vi "myRIO v1.0 Read I2C.vi"(4 "Keep Bus Busy":bool, 6 "Slave Address (7-bit)":u8, 7 "Timeout ms (1000)":i32=1000, 8 "Error In (No Error)":errorcluster, 9 "Bytes to Read":u32, 10 "Channel":T1, 11 "myRIO Ref In":T2) -> (0 "error out":errorcluster, 2 "Data Read":u8[](array[numeric]), 3 "myRIO Ref Out":T2)   [LabVIEW 2021]
uses:
  <vilib>/myRIO/Common/Instrument Driver Framework/Utilities/typedefs/myRIO v1.0 Reference.ctl
  <vilib>/myRIO/Common/Instrument Driver Framework/Utilities/typedefs/Generic FPGA Reference.ctl
  <vilib>/myRIO/Common/Instrument Driver Framework/myRIO v1.0/I2C/typedefs/I2C Channels Enum.ctl
  <vilib>/myRIO/Common/Instrument Driver Framework/myRIO v1.0/I2C/typedefs/I2C Channels FPGA Reference.ctl
  <vilib>/rvi/errors/niLvFpgaAdjustHostInterfaceError.vi
  <vilib>/rvi/interface/nirviReadWriteControl/nirviReadWriteControl.xnode
  <vilib>/rvi/interface/Simulation/niFpgaSimulationCallBeginRW.vi
  NiFpgaLv.dll
panel:
  # "This VI writes an array of data to the SPI Data Out register (SPIn.SPDO) and reads an array of data from the SPI Data In register (SPIn.SPDI) for a particular SPI channel (n). The data is written/read one value at a time. Please see Block Diagram for details."
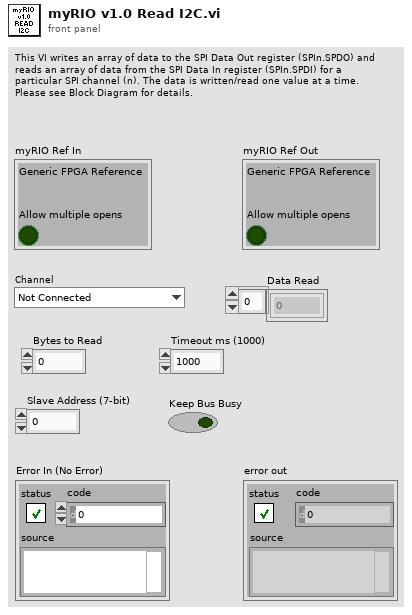
[diagram p1: front panel]
types:
  T1 = typedef "I2C Channels Enum.ctl" = enum16{"Not Connected", "A/I2C", "B/I2C", "I2C/I2C"}
  T2 = typedef "myRIO v1.0 Reference.ctl" = cluster{"Generic FPGA Reference":T3, "Allow multiple opens":bool}
  T3 = typedef "Generic FPGA Reference.ctl" = refnum<k20>
  T4 = typedef "I2C Channels FPGA Reference.ctl" = refnum<k20>
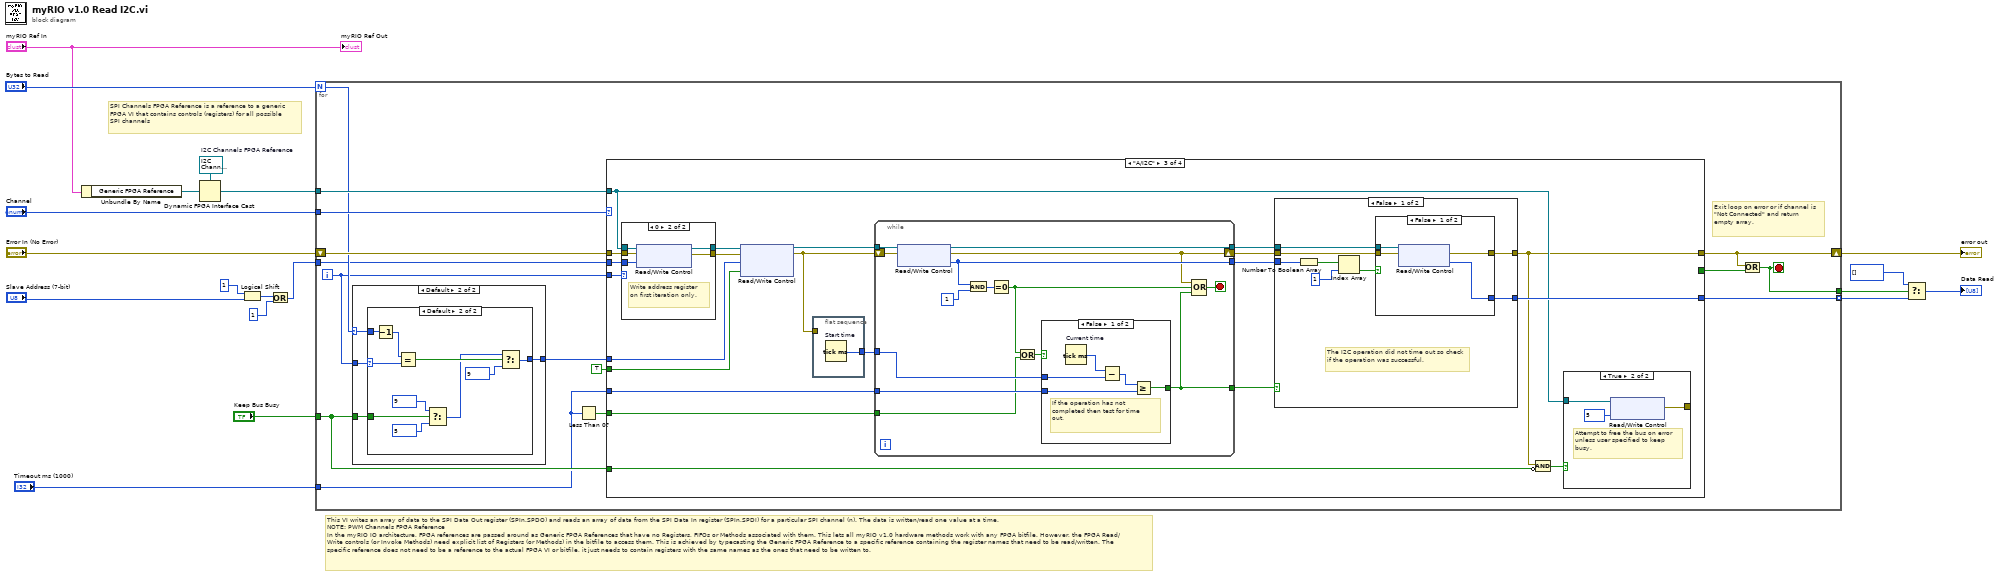
[diagram p0: block diagram]
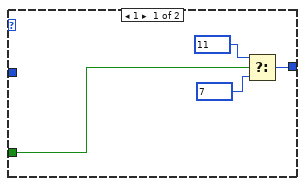
[diagram p2: hidden frame]
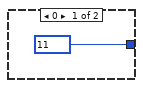
[diagram p3: hidden frame]
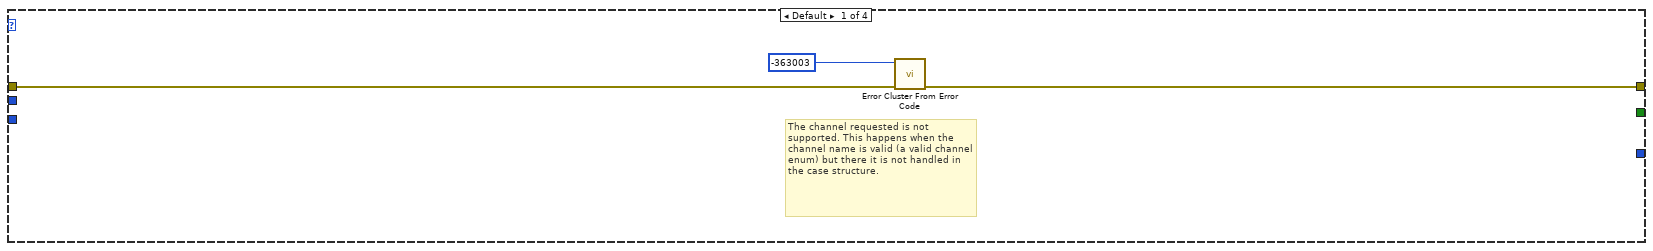
[diagram p4: hidden frame]
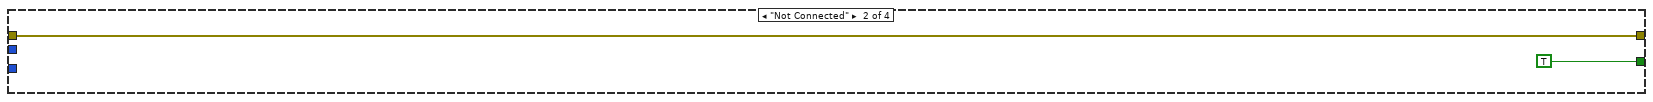
[diagram p5: hidden frame]
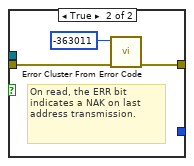
[diagram p6: hidden frame]
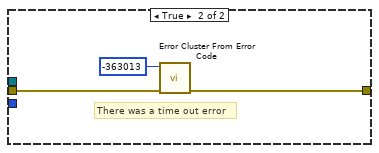
[diagram p7: hidden frame]
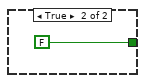
[diagram p10: hidden frame]
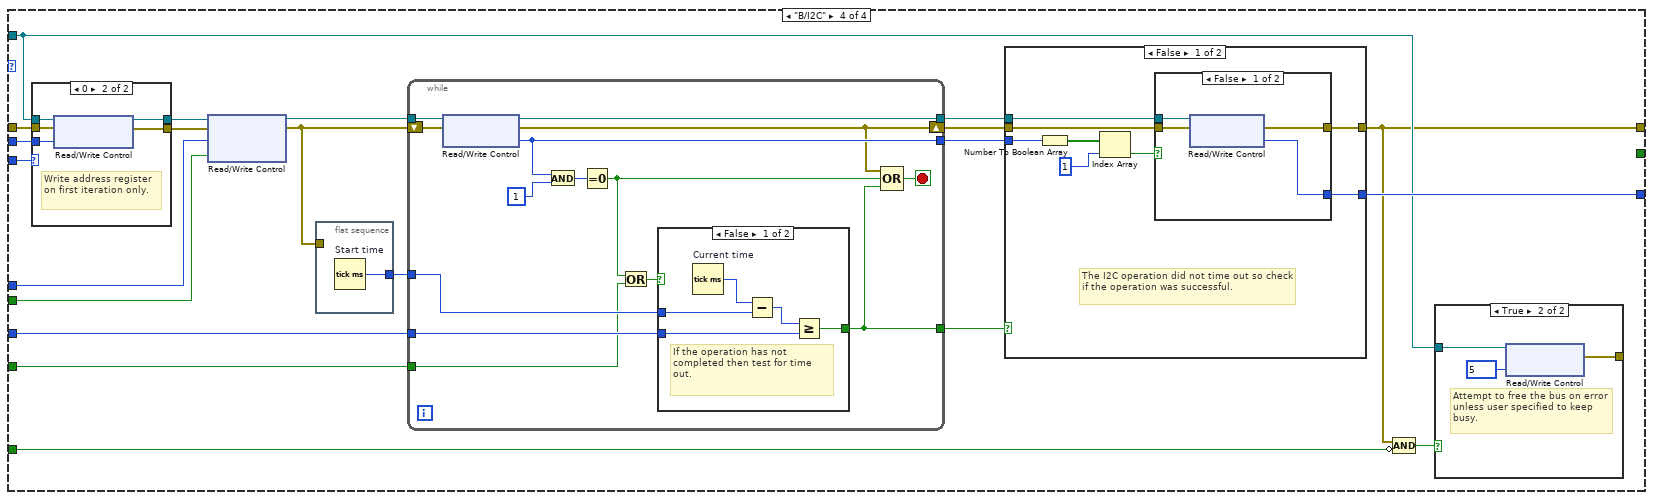
[diagram p11: hidden frame]
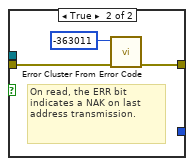
[diagram p12: hidden frame]
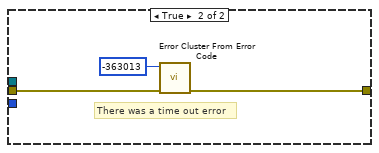
[diagram p13: hidden frame]
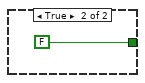
[diagram p16: hidden frame]
diagram:
  w17 = T4 refnum  # I2C Channels FPGA Reference
  # "This VI writes an array of data to the SPI Data Out register (SPIn.SPDO) and reads an array of data from the SPI Data In register (SPIn.SPDI) for a particular SPI channel (n). The data is written/read one value at a time.\nNOTE: PWM Channels FPGA Reference\nIn the myRIO IO architecture, FPGA references are passed around as Generic FPGA References that have no Registers, FIFOs or Methods associated with them. This lets all myRIO v1.0 hardware methods work with any FPGA bitfile. However, the FPGA Read/Write controls (or Invoke Methods) need explicit list of Registers (or Methods) in the bitfile to access them. This is achieved by typecasting the Generic FPGA Reference to a specific reference containing the register names that need to be read/written. The specific reference does not need to be a reference to the actual FPGA VI or bitfile, it just needs to contain registers with the same names as the ones that need to be written to."
  # "SPI Channels FPGA Reference is a reference to a generic FPGA VI that contains controls (registers) for all possible SPI channels"
  n1 = Unbundle By Name("myRIO Ref In") -> ("Generic FPGA Reference"=w1:T3)
  n2 = Dynamic FPGA Interface Cast(Session In=w17, Type=w1) -> (Session Out=w5:T4)
  n3 = Logical Shift(y=i8 1, x="Slave Address (7-bit)") -> (x << y=w16:u8)
  n4 = Or(x=w16, y=u8 1) -> (x .or. y?=w4:u8)
  n5 = for {
    N: "Bytes to Read" -> [w29]
    tunnel: "Channel" -> [w33]
    shift-right: [w24] -> w9
    shift-left: "Error In (No Error)" -> [w34]
    tunnel: w5 -> [w32]
    tunnel: [w28] -> w7 mode=indexing
    tunnel: [w22] -> w8
    tunnel: "Keep Bus Busy" -> [w25]
    tunnel: w4 -> [w27]
    tunnel: "Timeout ms (1000)" -> [w21]
    i -> [w26]
    stop <- w22 stop-if-true
    # "Exit loop on error or if channel is \"Not Connected\" and return empty array."
    n6 = case shown="Default" w29 {
      selector: w29 -> [_ w40]
      tunnel: [w38 w41] -> w30
      tunnel: w26 -> [_ w42]
      tunnel: w25 -> [w36 w39]
      frame 1 {
        n7 = Select(t=u8 11 ("y"), s=w36, f=u8 7 ("y")) -> (s? t:f=w38:u8)
      }
      frame Default {
        n8 = case shown="Default" w42 {
          selector: w42 -> [_ w51]
          tunnel: [u8 11 ("y") w49] -> w41
          tunnel: w40 -> [_ w53]
          tunnel: w39 -> [_ w46]
          frame 0 {
          }
          frame Default {
            n9 = Decrement(x=w53) -> (x-1=w52:i32)
            n10 = Equal?(x=w52, y=w51) -> (x = y?=w50:bool)
            n11 = Select(t=u8 9 ("y"), s=w46, f=u8 5 ("y")) -> (s? t:f=w45:u8)
            n12 = Select(t=w45, s=w50, f=u8 9 ("y")) -> (s? t:f=w49:u8)
          }
        }
      }
    }
    n13 = Less Than 0?(x=w21) -> (x < 0?=w20:bool)
    n14 = case shown="\"A/I2C\"" w33 {
      tunnel: w34 -> [w55 w58 w70 w140]
      tunnel: [w54 w58 w65 w135] -> w24
      tunnel: w32 -> [_ _ w67 w137]
      tunnel: w30 -> [_ _ w79 w149]
      tunnel: TRUE ("I2C0.GO") -> [_ _ w78 w148]
      tunnel: [_ _ w74 w144] -> w28
      tunnel: [_ TRUE _ _] -> w23
      tunnel: w27 -> [_ _ w69 w139]
      tunnel: w26 -> [_ _ w68 w138]
      tunnel: w25 -> [_ _ w66 w136]
      tunnel: w21 -> [_ _ w61 w131]
      tunnel: w20 -> [_ _ w60 w130]
      frame Default {
        # "The channel requested is not supported. This happens when the channel name is valid (a valid channel enum) but there it is not handled in the case structure."
        n15 = call <vilib>:"Error Cluster From Error Code.vi"("error in (no error)"=w55, "error code (0)"=-363003) -> ("error out"=w54:errorcluster)  [unwired: 7 in]
      }
      frame "Not Connected" {
      }
      frame "A/I2C" {
        n16 = case shown="0" w68 {
          tunnel: [w103 w108] -> w72
          tunnel: [w102 w107] -> w71
          tunnel: w67 -> [w103 w106]
          tunnel: w70 -> [w102 w105]
          tunnel: w69 -> [_ w104]
          frame Default {
          }
          frame 0 {
            # "Write address register on first iteration only."
            n17 = xnode "Read/Write Control"("FPGA VI Reference In"=w106, "error in"=w105, "I2C.A.ADDR"=w104) -> ("FPGA VI Reference Out"=w108:T4, "error out"=w107:errorcluster)
          }
        }
        n18 = xnode "Read/Write Control"("FPGA VI Reference In"=w72, "error in"=w71, "I2C.A.CNTL"=w79, "I2C.A.GO"=w78) -> ("FPGA VI Reference Out"=w77:T4, "error out"=w59:errorcluster)
        n19 = flat-sequence {
          tunnel: [w80] -> w63
          tunnel: w59 -> [_]
          frame #0 {
            n20 = Tick Count (ms) "Start time"() -> (millisecond timer value=w80:u32)
          }
        }
        n21 = while {
          tunnel: w77 -> [w121]
          shift-right: [w115] -> w76
          shift-left: w59 -> [w122]
          tunnel: [w117] -> w75
          tunnel: [w116] -> w73
          tunnel: w63 -> [w114]
          tunnel: [w113] -> w62
          tunnel: w61 -> [w112]
          tunnel: w60 -> [w110]
          stop <- w118 stop-if-true
          n22 = xnode "Read/Write Control"("FPGA VI Reference In"=w121, "error in"=w122) -> ("FPGA VI Reference Out"=w116:T4, "error out"=w115:errorcluster, "I2C.A.STAT"=w117:u8)
          n23 = And(x=w117, y=u8 1) -> (x .and. y?=w119:u8)
          n24 = Equal To 0?(x=w119) -> (x = 0?=w109:bool)
          n25 = Or(x=w109, y=w110) -> (x .or. y?=w111:bool)
          n26 = case shown="False" w111 {
            tunnel: w114 -> [w125 _]
            tunnel: [w124 FALSE] -> w113
            tunnel: w112 -> [w123 _]
            frame False {
              # "If the operation has not completed then test for time out."
              n27 = Tick Count (ms) "Current time"() -> (millisecond timer value=w126:u32)
              n28 = Subtract(x=w126, y=w125) -> (x-y=w127:u32)
              n29 = Greater Or Equal?(x=w127, y=w123) -> (x >= y?=w124:bool)
            }
            frame True {
            }
          }
          n30 = Compound Arithmetic op=OR(w115, w109, w113) -> (w118:bool)
        }
        n31 = case shown="False" w62 {
          tunnel: w76 -> [w88 w97]
          tunnel: w75 -> [w87 _]
          tunnel: [w83 _] -> w74
          tunnel: w73 -> [w82 _]
          tunnel: [w81 w96] -> w65
          frame False {
            # "The I2C operation did not time out so check if the operation was successful."
            n32 = Number To Boolean Array(number=w87) -> (Boolean array=w86:bool[])
            n33 = Index Array(array=w86, index=1) -> (element=w85:bool)
            n34 = case shown="False" w85 {
              tunnel: w88 -> [w90 w93]
              tunnel: [w91 w95] -> w81
              tunnel: [w92 _] -> w83
              tunnel: w82 -> [w89 _]
              frame False {
                n35 = xnode "Read/Write Control"("FPGA VI Reference In"=w89, "error in"=w90) -> ("error out"=w91:errorcluster, "I2C.A.DATI"=w92:u8)  [unwired: 1 out]
              }
              frame True {
                # "On read, the ERR bit indicates a NAK on last address transmission."
                n36 = call <vilib>:"Error Cluster From Error Code.vi"("error in (no error)"=w93, "error code (0)"=-363011) -> ("error out"=w95:errorcluster)  [unwired: 7 in]
              }
            }
          }
          frame True {
            # "There was a time out error"
            n37 = call <vilib>:"Error Cluster From Error Code.vi"("error in (no error)"=w97, "error code (0)"=-363013) -> ("error out"=w96:errorcluster)  [unwired: 7 in]
          }
        }
        n38 = Compound Arithmetic op=AND(w65, invert w66) -> (w64:bool)
        n39 = case shown="True" w64 {
          tunnel: w67 -> [_ w101]
          tunnel: [_ w99] -> _
          frame False {
          }
          frame True {
            # "Attempt to free the bus on error unless user specified to keep busy."
            n40 = xnode "Read/Write Control"("FPGA VI Reference In"=w101, "I2C.A.CNTL"=u8 5 ("I2C.C_0.CNTL")) -> ("error out"=w99:errorcluster)  [unwired: 1 in, 1 out]
          }
        }
      }
      frame "B/I2C" {
        n41 = case shown="0" w138 {
          tunnel: [w173 w178] -> w142
          tunnel: [w172 w177] -> w141
          tunnel: w137 -> [w173 w176]
          tunnel: w140 -> [w172 w175]
          tunnel: w139 -> [_ w174]
          frame Default {
          }
          frame 0 {
            # "Write address register on first iteration only."
            n42 = xnode "Read/Write Control"("FPGA VI Reference In"=w176, "error in"=w175, "I2C.B.ADDR"=w174) -> ("FPGA VI Reference Out"=w178:T4, "error out"=w177:errorcluster)
          }
        }
        n43 = xnode "Read/Write Control"("FPGA VI Reference In"=w142, "error in"=w141, "I2C.B.CNTL"=w149, "I2C.B.GO"=w148) -> ("FPGA VI Reference Out"=w147:T4, "error out"=w129:errorcluster)
        n44 = flat-sequence {
          tunnel: [w150] -> w133
          tunnel: w129 -> [_]
          frame #0 {
            n45 = Tick Count (ms) "Start time"() -> (millisecond timer value=w150:u32)
          }
        }
        n46 = while {
          tunnel: w147 -> [w191]
          shift-right: [w185] -> w146
          shift-left: w129 -> [w192]
          tunnel: [w187] -> w145
          tunnel: [w186] -> w143
          tunnel: w133 -> [w184]
          tunnel: [w183] -> w132
          tunnel: w131 -> [w182]
          tunnel: w130 -> [w180]
          stop <- w188 stop-if-true
          n47 = xnode "Read/Write Control"("FPGA VI Reference In"=w191, "error in"=w192) -> ("FPGA VI Reference Out"=w186:T4, "error out"=w185:errorcluster, "I2C.B.STAT"=w187:u8)
          n48 = And(x=w187, y=u8 1) -> (x .and. y?=w189:u8)
          n49 = Equal To 0?(x=w189) -> (x = 0?=w179:bool)
          n50 = Or(x=w179, y=w180) -> (x .or. y?=w181:bool)
          n51 = case shown="False" w181 {
            tunnel: w184 -> [w195 _]
            tunnel: [w194 FALSE] -> w183
            tunnel: w182 -> [w193 _]
            frame False {
              # "If the operation has not completed then test for time out."
              n52 = Tick Count (ms) "Current time"() -> (millisecond timer value=w196:u32)
              n53 = Subtract(x=w196, y=w195) -> (x-y=w197:u32)
              n54 = Greater Or Equal?(x=w197, y=w193) -> (x >= y?=w194:bool)
            }
            frame True {
            }
          }
          n55 = Compound Arithmetic op=OR(w185, w179, w183) -> (w188:bool)
        }
        n56 = case shown="False" w132 {
          tunnel: w146 -> [w158 w167]
          tunnel: w145 -> [w157 _]
          tunnel: [w153 _] -> w144
          tunnel: w143 -> [w152 _]
          tunnel: [w151 w166] -> w135
          frame False {
            # "The I2C operation did not time out so check if the operation was successful."
            n57 = Number To Boolean Array(number=w157) -> (Boolean array=w156:bool[])
            n58 = Index Array(array=w156, index=1) -> (element=w155:bool)
            n59 = case shown="False" w155 {
              tunnel: w158 -> [w160 w163]
              tunnel: [w161 w165] -> w151
              tunnel: [w162 _] -> w153
              tunnel: w152 -> [w159 _]
              frame False {
                n60 = xnode "Read/Write Control"("FPGA VI Reference In"=w159, "error in"=w160) -> ("error out"=w161:errorcluster, "I2C.B.DATI"=w162:u8)  [unwired: 1 out]
              }
              frame True {
                # "On read, the ERR bit indicates a NAK on last address transmission."
                n61 = call <vilib>:"Error Cluster From Error Code.vi"("error in (no error)"=w163, "error code (0)"=-363011) -> ("error out"=w165:errorcluster)  [unwired: 7 in]
              }
            }
          }
          frame True {
            # "There was a time out error"
            n62 = call <vilib>:"Error Cluster From Error Code.vi"("error in (no error)"=w167, "error code (0)"=-363013) -> ("error out"=w166:errorcluster)  [unwired: 7 in]
          }
        }
        n63 = Compound Arithmetic op=AND(w135, invert w136) -> (w134:bool)
        n64 = case shown="True" w134 {
          tunnel: w137 -> [_ w171]
          tunnel: [_ w169] -> _
          frame False {
          }
          frame True {
            # "Attempt to free the bus on error unless user specified to keep busy."
            n65 = xnode "Read/Write Control"("FPGA VI Reference In"=w171, "I2C.B.CNTL"=u8 5 ("I2C.C_0.CNTL")) -> ("error out"=w169:errorcluster)  [unwired: 1 in, 1 out]
          }
        }
      }
    }
    n66 = Or(x=w24, y=w23) -> (x .or. y?=w22:bool)
  }
  "error out" <- w9
  n67 = Select(t=u8[] [], s=w8, f=w7) -> (s? t:f=→"Data Read":u8[])
  "myRIO Ref Out" <- "myRIO Ref In"
